vi "Configure Digital IQ Data.vi"(0 "VISA resource name":refnum<visa-resource-name>, 1 "I Gain (0 percent)":dbl, 2 "Enable I Negation (F:Disable)":bool, 5 "Enable Q Negation (F:Disable)":bool, 7 "Q Gain (0 percent)":dbl, 9 "Enable I/Q Swap (F:Disable)":bool, 11 "error in (no error)":errorcluster, 12 "I/Q Polarity (0: Positive)":u16(ring) items=["Positive", "Negative"]) -> (4 "VISA resource name out":refnum<visa-resource-name>, 15 "error out":errorcluster)   [LabVIEW 2012, in "Agilent PSG MXG Series.lvlib"]
doc: "Configures I and Q data.\n\n<B>Notes:</B>\n(1) This VI is valid only in E8267D that installs <B>Option 601</B> or <B>Option 602</B> (Internal baseband generator), and <B>Option 003</B> (PSG digital output connectivity with N5102A) or <B>Option 004</B> (PSG digital input connectivity with N5102A)."
uses:
  <instrlib>/Agilent PSG MXG Series/Agilent PSG MXG Series.lvlib
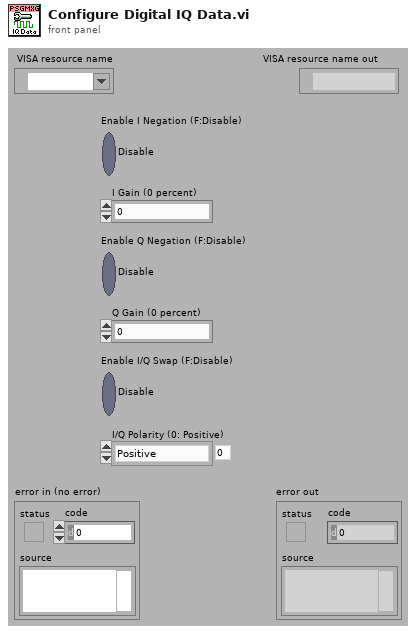
[diagram p1: front panel]
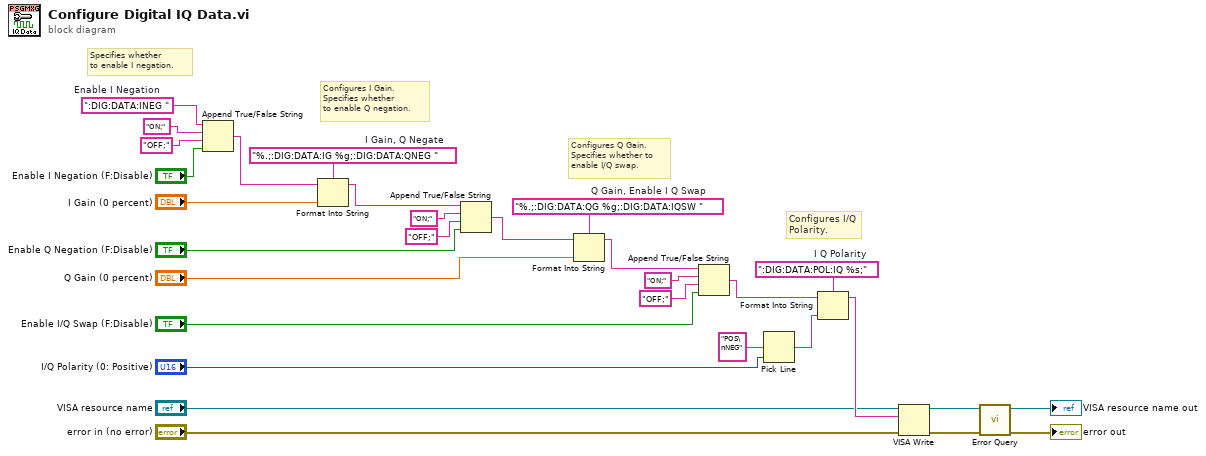
[diagram p0: block diagram]
diagram:
  w11 = ":DIG:DATA:POL:IQ %s;"  # I Q Polarity
  w18 = "%.;:DIG:DATA:QG %g;:DIG:DATA:IQSW "  # Q Gain, Enable I Q Swap
  w25 = "%.;:DIG:DATA:IG %g;:DIG:DATA:QNEG "  # I Gain, Q Negate
  w30 = ":DIG:DATA:INEG "  # Enable I Negation
  # "Configures I/Q\nPolarity."
  # "Configures Q Gain.\nSpecifies whether to\nenable I/Q swap."
  # "Configures I Gain.\nSpecifies whether\nto enable Q negation."
  # "Specifies whether\nto enable I negation."
  n1 = Append True/False String(1:"Enable I Negation (F:Disable)", 2:"OFF;" ("false string"), 3:"ON;" ("true string"), 4:w30) -> (0:w26:string)
  n2 = Format Into String(format string=w25, initial string=w26, "I Gain (0 percent)") -> (resulting string=w23:string)  [unwired: 1 in, 1 out]
  n3 = Append True/False String(1:"Enable Q Negation (F:Disable)", 2:"OFF;" ("false string"), 3:"ON;" ("true string"), 4:w23) -> (0:w19:string)
  n4 = Format Into String(format string=w18, initial string=w19, "Q Gain (0 percent)") -> (resulting string=w16:string)  [unwired: 1 in, 1 out]
  n5 = Append True/False String(1:"Enable I/Q Swap (F:Disable)", 2:"OFF;" ("false string"), 3:"ON;" ("true string"), 4:w16) -> (0:w12:string)
  n6 = Pick Line(multi-line string="POS\nNEG", line index="I/Q Polarity (0: Positive)") -> (output string=w10:string)  [unwired: 1 out]
  n7 = Format Into String(format string=w11, initial string=w12, w10) -> (resulting string=w7:string)  [unwired: 1 in, 1 out]
  n8 = VISA Write(VISA resource name="VISA resource name", write buffer=w7, error in (no error)="error in (no error)") -> (VISA resource name out=w6:refnum<visa-resource-name>, error out=w5:errorcluster)  [unwired: 1 out]
  n9 = call <instrlib>:"Error Query.vi"("error in (no error)"=w5, "VISA resource name"=w6) -> ("error out"=→"error out":errorcluster, "VISA resource name out"=→"VISA resource name out":refnum<visa-resource-name>)  [unwired: 8 out]
